vi "Find Dynamic Node Details.vi"(8 "error in":errorcluster, 10 "Parent Node":string, 11 "Node In":refnum<k20>) -> (0 "error out":errorcluster, 2 "Dynamic Page Properties":T1[](array[typedef]))   [LabVIEW 2026, in "NIVS_CDEW_MetaDataObj.lvclass"]
uses:
  Types/Page Properties.ctl
  Types/Page Types.ctl
  NIVS_CDEW_MetaDataObj.lvclass
  NIVS_CDEW_MetaDataObj.lvclass/NIVS_CDEW_MetaDataObj.ctl
  <resource>/objmgr/DOMUserDefRef.rc
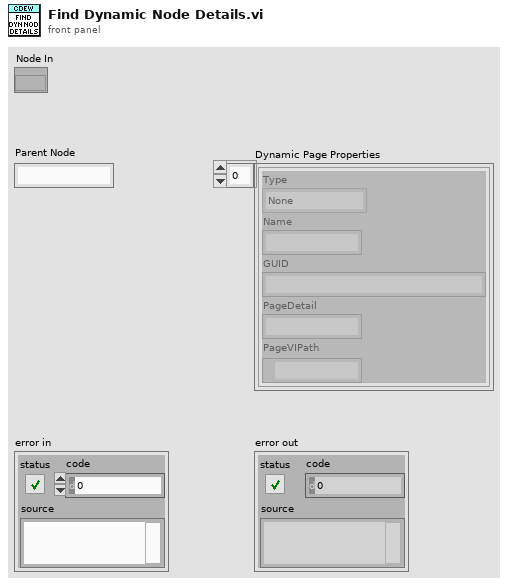
[diagram p1: front panel]
types:
  T1 = typedef "NIVS_CDEW_MetaDataObj.lvclass/Page Properties.ctl" = cluster{"Type":T2, "Name":string, "GUID":string, "PageDetail":string, "PageVIPath":path}
  T2 = typedef "NIVS_CDEW_MetaDataObj.lvclass/Page Types.ctl" = enum16{"None", "CustomDevice", "Channel", "Waveform", "Section", "DynamicChannel", "DynamicWaveform", "DynamicSection"}
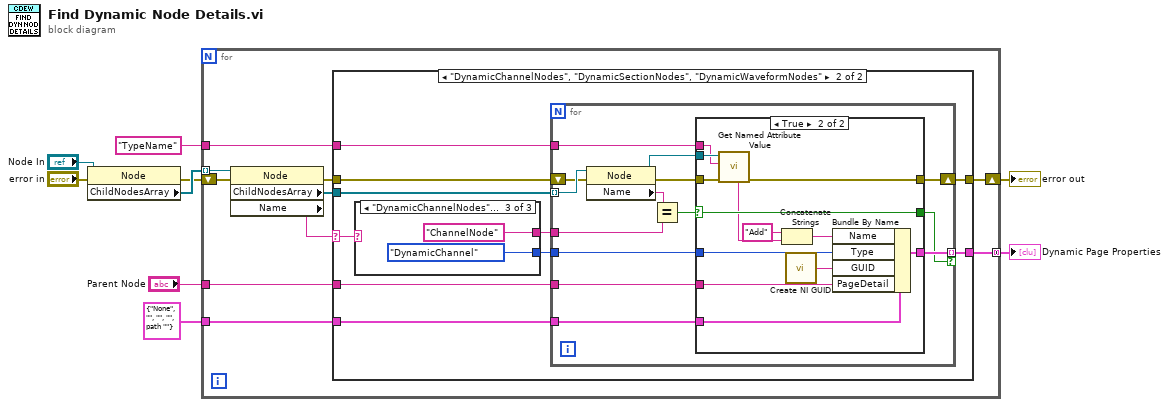
[diagram p0: block diagram]
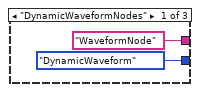
[diagram p3: hidden frame]
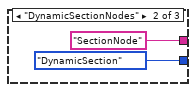
[diagram p4: hidden frame]
diagram:
  n1 = property class="Node"(reference="Node In", error in="error in") -> (error out=w6:errorcluster, "ChildNodesArray"=w9:refnum<k20>[])  [unwired: 1 out]
  n2 = for {
    tunnel: w9 -> [w19] mode=indexing
    shift-right: [w15] -> w4
    shift-left: w6 -> [w17]
    tunnel: "TypeName" -> [w14]
    tunnel: [w12] -> w2 mode=concatenating
    tunnel: T1 {"Type"=enum."None", "Name"="", "GUID"="", "PageDetail"="", "PageVIPath"=path ""} ("Page Properties") -> [w11]
    tunnel: "Parent Node" -> [w10]
    n3 = property class="Node"(reference=w19, error in=w17) -> (error out=w16:errorcluster, "ChildNodesArray"=w18:refnum<k20>[], "Name"=w13:string)  [unwired: 1 out]
    n4 = case shown="\"DynamicChannelNodes\", \"DynamicSectionNodes\", \"DynamicWaveformNodes\"" w13 {
      selector: w13 -> [_ w26]
      tunnel: w18 -> [_ w30]
      tunnel: w16 -> [w20 w29]
      tunnel: [w20 w27] -> w15
      tunnel: w14 -> [_ w28]
      tunnel: [_ w24] -> w12
      tunnel: w11 -> [_ w22]
      tunnel: w10 -> [_ w21]
      frame Default {
      }
      frame "DynamicChannelNodes", "DynamicSectionNodes", "DynamicWaveformNodes" {
        n5 = case shown="\"DynamicChannelNodes\", Default" w26 {
          tunnel: ["WaveformNode" "SectionNode" "ChannelNode"] -> w25
          tunnel: [Page_Types."DynamicWaveform" ("Type") Page_Types."DynamicSection" ("Type") Page_Types."DynamicChannel" ("Type")] -> w23
          frame "DynamicWaveformNodes" {
          }
          frame "DynamicSectionNodes" {
          }
          frame "DynamicChannelNodes", Default {
          }
        }
        n6 = for {
          tunnel: w30 -> [w50] mode=indexing
          shift-right: [w43] -> w27
          shift-left: w29 -> [w48]
          tunnel: w25 -> [w42]
          tunnel: w28 -> [w44]
          tunnel: [w41] -> w24 mode=indexing if=w40
          tunnel: w23 -> [w39]
          tunnel: w22 -> [w38]
          tunnel: w21 -> [w37]
          n7 = property class="Node"(reference=w50, error in=w48) -> (reference out=w45:refnum<k20>, error out=w46:errorcluster, "Name"=w49:string)
          n8 = Equal?(x=w42, y=w49) -> (x = y?=w47:bool)
          n9 = case shown="True" w47 {
            selector: w47 -> [_ w59]
            tunnel: w46 -> [w51 w64]
            tunnel: w45 -> [_ w63]
            tunnel: w44 -> [_ w62]
            tunnel: [w51 w61] -> w43
            tunnel: [_ w60] -> w41
            tunnel: [_ w59] -> w40
            tunnel: w39 -> [_ w58]
            tunnel: w38 -> [_ w56]
            tunnel: w37 -> [_ w52]
            frame False {
            }
            frame True {
              n10 = call "Get Named Attribute Value.vi"("error in"=w64, "Attribute Name"=w62, "Node In"=w63) -> ("error out"=w61:errorcluster, "Attribute Value"=w55:string)  [unwired: 5 in, 2 out]
              n11 = Concatenate Strings("Add" ("string"), w55) -> (w54:string)
              n12 = call <vilib>:"Create NI GUID.vi"() -> ("NI GUID"=w57:string)
              n13 = Bundle By Name(cluster=w56, "Name"=w54, "Type"=w58, "GUID"=w57, "PageDetail"=w52) -> (w60:T1)
            }
          }
        }
      }
    }
  }
  "error out" <- w4
  "Dynamic Page Properties" <- w2
